vi "adjust.vi"(8 "error in (no error)":errorcluster, 11 "LightSourceAN191011Chameleon in":refnum<class "LightSourceAN191011Chameleon.lvclass">) -> (0 "error out":errorcluster, 3 "LightSourceAN191011Chameleon out":refnum<class "LightSourceAN191011Chameleon.lvclass">)   [LabVIEW 2010, in "LightSourceAN191011Chameleon.lvclass"]
uses:
  LightSourceAN191011Chameleon.lvclass
  LightSourceAN191011Chameleon.lvclass/LightSourceAN191011Chameleon.ctl
  common/classes/ErrorController/ErrorController/class_data.vi
  common/classes/ErrorController/ErrorController/ErrorController.lvclass
panel:
  out "pulsing":bool
  in  "shutter":bool
  in  "wavelength":i32(slide) scale=680.0..1080.0
  in  "initialise?":bool
  in  "switch off":bool
  in  "stop":bool
  out "get wavelength":dbl[unit](slide)
  out "power":dbl[unit](slide) scale=0.0..4.0
  in  "alignment mode":bool
  # "laser"
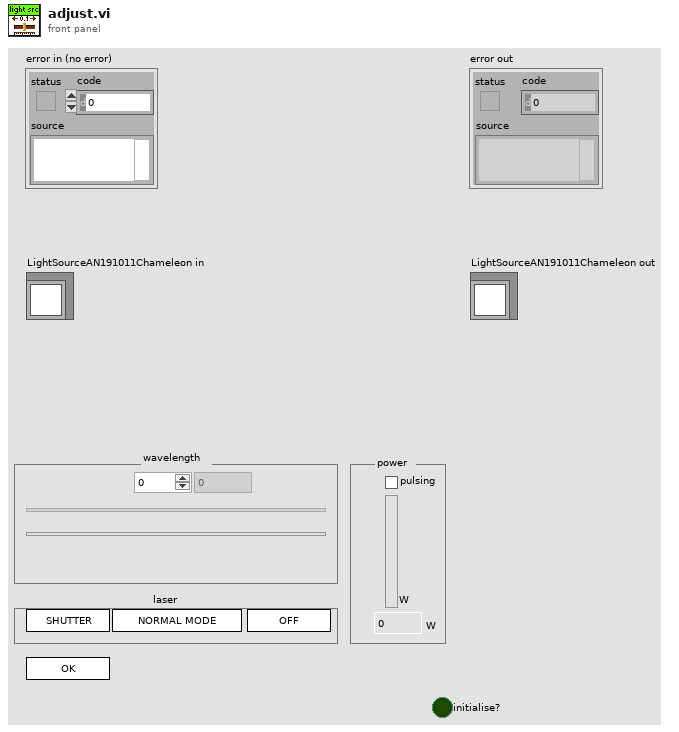
[diagram p1: front panel]
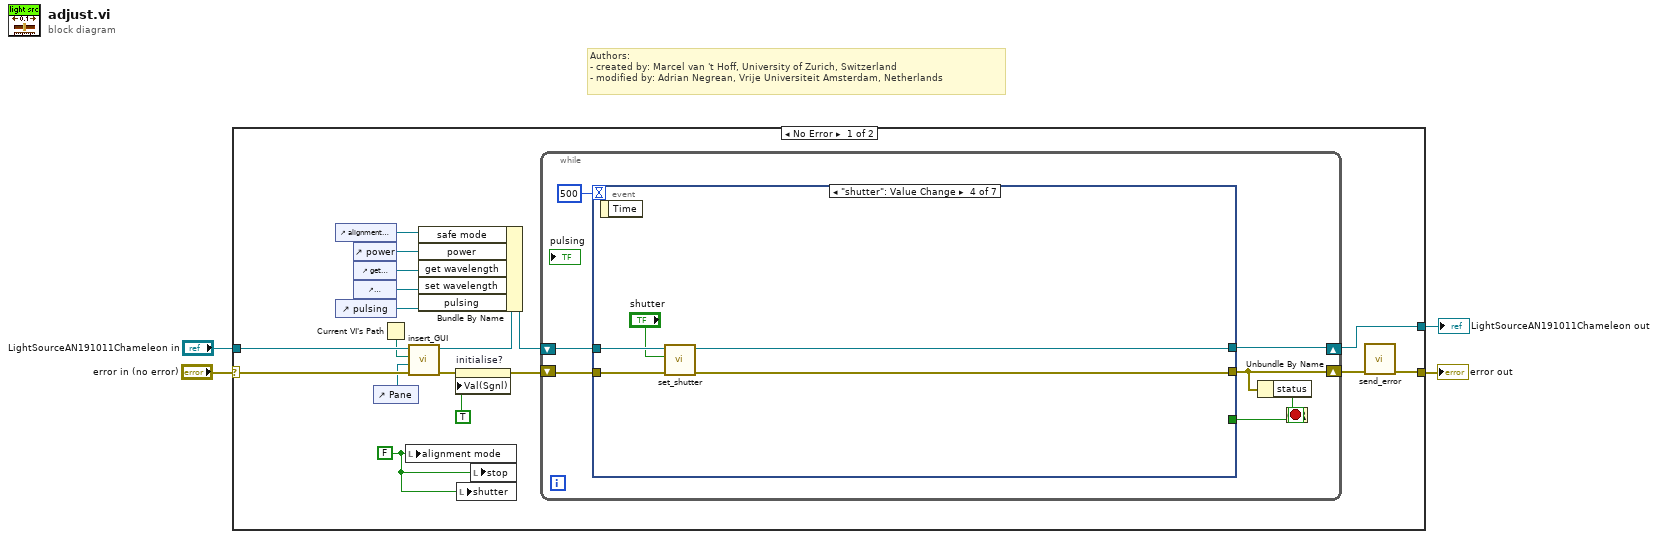
[diagram p0: block diagram]
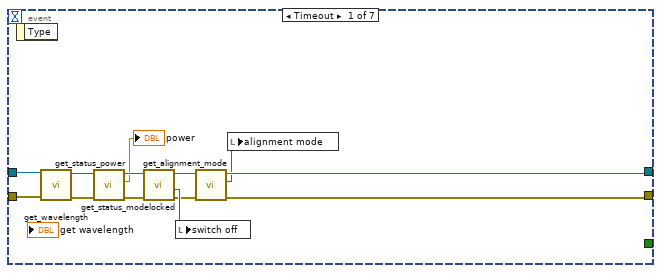
[diagram p2: hidden frame]
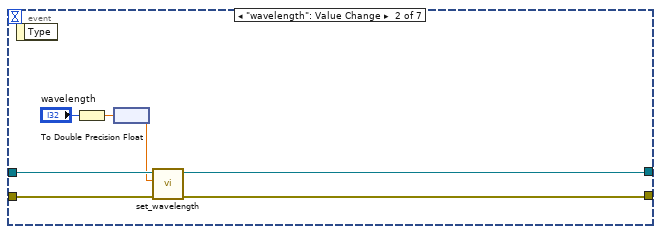
[diagram p3: hidden frame]
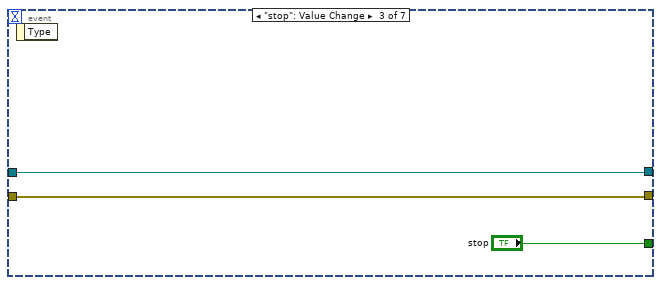
[diagram p4: hidden frame]
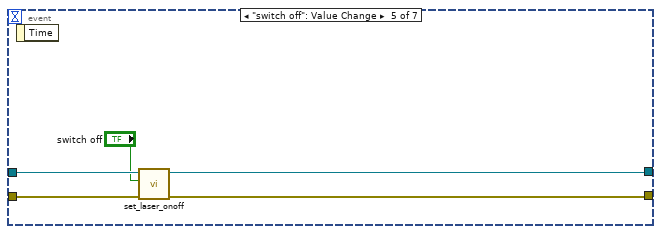
[diagram p5: hidden frame]
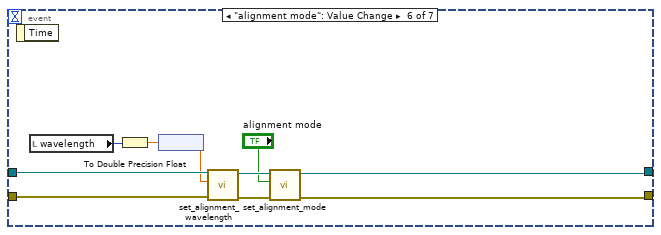
[diagram p6: hidden frame]
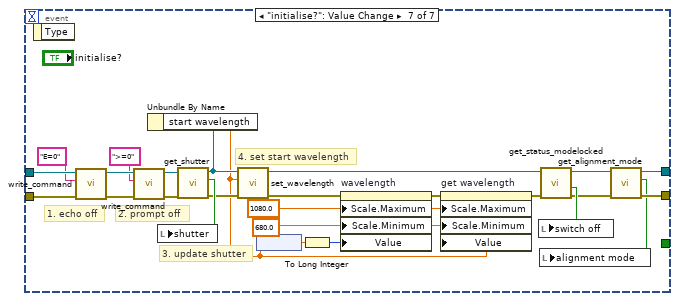
[diagram p7: hidden frame]
diagram:
  # "Authors: \n- created by: Marcel van 't Hoff, University of Zurich, Switzerland\n- modified by: Adrian Negrean, Vrije Universiteit Amsterdam, Netherlands"
  n1 = case shown="No Error" "error in (no error)" {
    selector: "error in (no error)" -> [w16 w101]
    tunnel: [w9 w101] -> w3
    tunnel: "LightSourceAN191011Chameleon in" -> [w18 w100]
    tunnel: [w8 w100] -> w1
    frame No Error {
      w5 = FALSE ("alignment mode")
      n2 = control-ref of="alignment mode"() -> (w21:refnum<vi>)
      n3 = control-ref of="pulsing"() -> (w6:refnum<vi>)
      n4 = control-ref of="power"() -> (w20:refnum<vi>)
      n5 = control-ref of="get wavelength"() -> (w19:refnum<vi>)
      n6 = control-ref of="wavelength"() -> (w7:refnum<vi>)
      n7 = control-ref of="Pane"() -> (w14:refnum<vi>)
      n8 = Current VI's Path() -> (path=w15:path)
      n9 = local write "alignment mode"(w5) -> ()
      n10 = call-dynamic "insert_GUI.vi"("error in (no error)"=w16, "Pane"=w14, "VI path"=w15, "GenericComponent in"=w18) -> ("error out"=w13:errorcluster, "GenericComponent out"=w17:refnum<class "LightSourceAN191011Chameleon.lvclass">)  [unwired: 6 in]
      n11 = Bundle By Name(cluster=w17, "safe mode"=w21, "power"=w20, "get wavelength"=w19, "set wavelength"=w7, "pulsing"=w6) -> (w22:refnum<class "LightSourceAN191011Chameleon.lvclass">)
      n12 = property on="initialise?" class="Bool (strict)"(error in=w13, "Val(Sgnl)"=TRUE ("Value (Signaling)")) -> (error out=w12:errorcluster)  [unwired: 1 in, 1 out]
      n13 = local write "shutter"(w5) -> ()
      n14 = local write "stop"(w5) -> ()
      n15 = while {
        shift-right: [w27] -> w10
        shift-left: w12 -> [w29]
        shift-right: [w24] -> w8
        shift-left: w22 -> [w30]
        stop <- w25 stop-if-true
        n16 = event shown="[3] \"shutter\": Value Change" {
          selector: _ -> [_ _ _ _ _ _ _]
          dyn-events: _ -> [_ _ _ _ _ _ _]
          timeout: 500 -> [_ _ _ _ _ _ _]
          tunnel: w30 -> [w43 w50 w52 w58 w63 w73 w99]
          tunnel: w29 -> [w42 w49 w51 w57 w62 w72 w98]
          tunnel: [w35 w45 w52 w55 w60 w65 w77] -> w24
          tunnel: [w33 w44 w51 w54 w59 w64 w75] -> w27
          tunnel: [_ _ "stop" _ _ _ _] -> w23
          event Timeout {
            n17 = event-data() -> ()  [unwired: 1 in, 1 out]
            n18 = call-dynamic "get_wavelength.vi"("error in (no error)"=w42, "LightSourceAN191011Chameleon in"=w43) -> ("error out"=w40:errorcluster, "LightSourceAN191011Chameleon out"=w41:refnum<class "LightSourceAN191011Chameleon.lvclass">)  [unwired: 7 in, 1 out]
            n19 = call-dynamic "get_status_power.vi"("error in (no error)"=w40, "LightSourceAN191011Chameleon in"=w41) -> ("error out"=w38:errorcluster, "output power"=→"power":dbl[unit], "LightSourceAN191011Chameleon out"=w39:refnum<class "LightSourceAN191011Chameleon.lvclass">)  [unwired: 7 in]
            n20 = call-dynamic "get_status_modelocked.vi"("error in (no error)"=w38, "LightSourceAN191011Chameleon in"=w39) -> ("error out"=w34:errorcluster, "Emission"=w37:bool, "LightSourceAN191011Chameleon out"=w36:refnum<class "LightSourceAN191011Chameleon.lvclass">)  [unwired: 6 in, 1 out]
            n21 = local write "switch off"(w37) -> ()
            n22 = call-dynamic "get_alignment_mode.vi"("error in (no error)"=w34, "LightSourceAN191011Chameleon in"=w36) -> ("error out"=w33:errorcluster, "alignment mode?"=w32:bool, "LightSourceAN191011Chameleon out"=w35:refnum<class "LightSourceAN191011Chameleon.lvclass">)  [unwired: 7 in]
            n23 = local write "alignment mode"(w32) -> ()
          }
          event "wavelength": Value Change {
            n24 = event-data() -> ()  [unwired: 1 in, 1 out]
            n25 = To Double Precision Float(number="wavelength") -> (double precision float=w48:dbl)
            n26 = node(w48) -> (w46:dbl[unit])
            n27 = call-dynamic "set_wavelength.vi"("error in (no error)"=w49, "wavelength in"=w46, "LightSourceAN191011Chameleon in"=w50) -> ("error out"=w44:errorcluster, "LightSourceAN191011Chameleon out"=w45:refnum<class "LightSourceAN191011Chameleon.lvclass">)  [unwired: 7 in]
          }
          event "stop": Value Change {
            n28 = event-data() -> ()  [unwired: 1 in, 1 out]
          }
          event "shutter": Value Change {
            n29 = event-data() -> ()  [unwired: 1 in, 1 out]
            n30 = call-dynamic "set_shutter.vi"("error in (no error)"=w57, "shutter open?"="shutter", "LightSourceAN191011Chameleon in"=w58) -> ("error out"=w54:errorcluster, "LightSourceAN191011Chameleon out"=w55:refnum<class "LightSourceAN191011Chameleon.lvclass">)  [unwired: 6 in, 1 out]
          }
          event "switch off": Value Change {
            n31 = event-data() -> ()  [unwired: 1 in, 1 out]
            n32 = call-dynamic "set_laser_onoff.vi"("error in (no error)"=w62, "laser on?"="switch off", "LightSourceAN191011Chameleon in"=w63) -> ("error out"=w59:errorcluster, "LightSourceAN191011Chameleon out"=w60:refnum<class "LightSourceAN191011Chameleon.lvclass">)  [unwired: 7 in]
          }
          event "alignment mode": Value Change {
            n33 = event-data() -> ()  [unwired: 1 in, 1 out]
            n34 = local read "wavelength"() -> (w71:i32)
            n35 = To Double Precision Float(number=w71) -> (double precision float=w70:dbl)
            n36 = node(w70) -> (w69:dbl[unit])
            n37 = call-dynamic "set_alignment_wavelength.vi"("error in (no error)"=w72, "wavelength in"=w69, "LightSourceAN191011Chameleon in"=w73) -> ("error out"=w67:errorcluster, "LightSourceAN191011Chameleon out"=w68:refnum<class "LightSourceAN191011Chameleon.lvclass">)  [unwired: 7 in]
            n38 = call-dynamic "set_alignment_mode.vi"("error in (no error)"=w67, "alignment mode?"="alignment mode", "LightSourceAN191011Chameleon in"=w68) -> ("error out"=w64:errorcluster, "LightSourceAN191011Chameleon out"=w65:refnum<class "LightSourceAN191011Chameleon.lvclass">)  [unwired: 7 in]
          }
          event "initialise?": Value Change {
            w82 = 680.0 ("Scale.Range:Minimum")
            w83 = 1080.0 ("Scale.Range:Maximum")
            # "4. set start wavelength"
            # "3. update shutter"
            # "2. prompt off"
            # "1. echo off"
            n39 = event-data() -> ()  [unwired: 1 in, 1 out]
            n40 = call-dynamic "write_command.vi"("error in (no error)"=w98, "string to write"="E=0", "LightSourceAN191011Chameleon in"=w99) -> ("error out"=w95:errorcluster, "LightSourceAN191011Chameleon out"=w96:refnum<class "LightSourceAN191011Chameleon.lvclass">)  [unwired: 6 in, 1 out]
            n41 = call-dynamic "write_command.vi"("error in (no error)"=w95, "string to write"=">=0", "LightSourceAN191011Chameleon in"=w96) -> ("error out"=w92:errorcluster, "LightSourceAN191011Chameleon out"=w93:refnum<class "LightSourceAN191011Chameleon.lvclass">)  [unwired: 6 in, 1 out]
            n42 = call-dynamic "get_shutter.vi"("error in (no error)"=w92, "LightSourceAN191011Chameleon in"=w93) -> ("error out"=w89:errorcluster, "shutter status"=w91:bool, "LightSourceAN191011Chameleon out"=w90:refnum<class "LightSourceAN191011Chameleon.lvclass">)  [unwired: 7 in]
            n43 = Unbundle By Name(w90) -> ("start wavelength"=w81:dbl[unit])
            n44 = local write "shutter"(w91) -> ()
            n45 = call-dynamic "set_wavelength.vi"("error in (no error)"=w89, "wavelength in"=w81, "LightSourceAN191011Chameleon in"=w90) -> ("error out"=w85:errorcluster, "LightSourceAN191011Chameleon out"=w88:refnum<class "LightSourceAN191011Chameleon.lvclass">)  [unwired: 7 in]
            n46 = node(w81) -> (w80:dbl)
            n47 = To Long Integer(number=w80) -> (32bit integer=w79:i32)
            n48 = property on="wavelength" class="Slide (strict)"(error in=w85, "Scale.Maximum"=w83, "Scale.Minimum"=w82, "Value"=w79) -> (error out=w84:errorcluster)  [unwired: 1 in, 1 out]
            n49 = property on="get wavelength" class="Slide (strict)"(error in=w84, "Scale.Maximum"=w83, "Scale.Minimum"=w82, "Value"=w81) -> (error out=w87:errorcluster)  [unwired: 1 in, 1 out]
            n50 = call-dynamic "get_status_modelocked.vi"("error in (no error)"=w87, "LightSourceAN191011Chameleon in"=w88) -> ("error out"=w76:errorcluster, "Emission"=w86:bool, "LightSourceAN191011Chameleon out"=w78:refnum<class "LightSourceAN191011Chameleon.lvclass">)  [unwired: 6 in, 1 out]
            n51 = local write "switch off"(w86) -> ()
            n52 = call-dynamic "get_alignment_mode.vi"("error in (no error)"=w76, "LightSourceAN191011Chameleon in"=w78) -> ("error out"=w75:errorcluster, "alignment mode?"=w74:bool, "LightSourceAN191011Chameleon out"=w77:refnum<class "LightSourceAN191011Chameleon.lvclass">)  [unwired: 7 in]
            n53 = local write "alignment mode"(w74) -> ()
          }
        }
        n54 = Unbundle By Name(w27) -> ("status"=w28:bool)
        n55 = Or(x=w28, y=w23) -> (x .or. y?=w25:bool)
      }
      n56 = call "send_error.vi"("error in (no error)"=w10) -> ("error out"=w9:errorcluster)  [unwired: 10 in]
    }
    frame Error {
    }
  }
  "error out" <- w3
  "LightSourceAN191011Chameleon out" <- w1
